vi "SPD.Measurments Single Point.vi"(5 "Current Progress":refnum<vi>, 6 "Overall Progress":refnum<vi>, 7 "Continue":refnum<vi>, 8 "Error In":errorcluster, 11 "SPD.Stand Ctrl in":T1={"spdDeviceSession"={"spdRef"=0, "connected"=FALSE, "spdName"="", "specification"={"diod case"=enum."default", "type"=enum."Unknown", "frequency"=enum."Unknown"}, "hidSPD.Controller"={"TSet"=0.0, "HV_bias"=0.0, "DDS_stb_code"=0}, "hidSPD.Sturtup Values"={"TSet"=0.0, "HV_bias"=0.0, "DDS_stb_code"=0}}, "DevBSession"={"DevBRef"="", "connected"=FALSE}, "FreqCSession"={"FreqCRef"="", "timeout"=0.0, "Gate"=0.0, "connected"=FALSE}, "8164BSession"={"Connection ID"=refnum, "Connected"=FALSE, "Info"="", "Slots Info"=[]}, "LeCroySession"={"LeCroySession"="", "connected"=FALSE}, "Events"={"DCRTest"=refnum, "Stop"=refnum}, "configFile"={"configFile ref"=refnum, "configFile path"=path "", "equipmentFile ref"=refnum}, "SPD.Meas Grid"={"DateTime"="", "DT"=[], "Insensitivity"=[], "Temprature"=[], "Stb_code"=[], "HV_Bias"=[]}, "SPD.Queues"={"state queue"=refnum}, "Console"=refnum} {"spdDeviceSession"."hidSPD.Sturtup Values"."HV_bias" format="%#_6p, V"; "spdDeviceSession"."hidSPD.Sturtup Values"."TSet" format="%#_6p, DegC"; "spdDeviceSession"."hidSPD.Controller"."HV_bias" format="%#_6p, V"; "spdDeviceSession"."hidSPD.Controller"."TSet" format="%#_6p, DegC"}) -> (0 "Error Out":errorcluster, 2 "pass":bool, 3 "SPD.Stand Ctrl out":T1={"spdDeviceSession"={"spdRef"=0, "connected"=FALSE, "spdName"="", "specification"={"diod case"=enum."default", "type"=enum."Unknown", "frequency"=enum."Unknown"}, "hidSPD.Controller"={"TSet"=0.0, "HV_bias"=0.0, "DDS_stb_code"=0}, "hidSPD.Sturtup Values"={"TSet"=0.0, "HV_bias"=0.0, "DDS_stb_code"=0}}, "DevBSession"={"DevBRef"="", "connected"=FALSE}, "FreqCSession"={"FreqCRef"="", "timeout"=0.0, "Gate"=0.0, "connected"=FALSE}, "8164BSession"={"Connection ID"=refnum, "Connected"=FALSE, "Info"="", "Slots Info"=[]}, "LeCroySession"={"LeCroySession"="", "connected"=FALSE}, "Events"={"DCRTest"=refnum, "Stop"=refnum}, "configFile"={"configFile ref"=refnum, "configFile path"=path "", "equipmentFile ref"=refnum}, "SPD.Meas Grid"={"DateTime"="", "DT"=[], "Insensitivity"=[], "Temprature"=[], "Stb_code"=[], "HV_Bias"=[]}, "SPD.Queues"={"state queue"=refnum}, "Console"=refnum} {"spdDeviceSession"."hidSPD.Sturtup Values"."HV_bias" format="%#_6p, V"; "spdDeviceSession"."hidSPD.Sturtup Values"."TSet" format="%#_6p, DegC"; "spdDeviceSession"."hidSPD.Controller"."HV_bias" format="%#_6p, V"; "spdDeviceSession"."hidSPD.Controller"."TSet" format="%#_6p, DegC"})   [LabVIEW 2018]
uses:
  Instruments/KC705 DevBoard/typedefs/DevB.Session.ctl
  Instruments/KeySight 53230A/typedefs/FreqC.Session.ctl
  Instruments/KeySight 8164B/KeySight 8164B LAN InstrLib/typedefs/KeySight 8164B control.ctl
  Instruments/KeySight 8164B/KeySight 8164B LAN InstrLib.lvlib
  Instruments/LeCroy SDA830/typedefs/LeCroy.Session.ctl
  typedefs/SPD.Events.ctl
  <vilib>/Utility/config.llb/Config Data RefNum.ctl
  <vilib>/Utility/config.llb/NI_LVConfig.lvlib
  ConfigFile/SPD.Config File ctrl.ctl
  typedefs/SPD.Meas Grid.ctl
  typedefs/SPD.Stand state.ctl
  typedefs/SPD.Queues.ctl
  Instruments/SPD HID Interface/hidSPDLibForLabView/LibVIs/hidSPD Controls/hidSPD Controller.ctl
  Instruments/SPD HID Interface/hidSPDLibForLabView/hidSPDLibForLabView.lvlib
  Instruments/SPD HID Interface/hidSPDLibForLabView/LibVIs/hidSPD Controls/hidSPD SPD Type.ctl
  Instruments/SPD HID Interface/hidSPDLibForLabView/LibVIs/hidSPD Controls/hidSPD Device Session.ctl
  typedefs/SPD.Stand Ctrl.ctl
  Instruments/SPD HID Interface/hidSPDLibForLabView/LibVIs/hidSPD Controls/hidSPD SPD Diod Case.ctl
  Instruments/SPD HID Interface/hidSPDLibForLabView/LibVIs/hidSPD Controls/hidSPD.STB Frequency.ctl
  Instruments/SPD HID Interface/hidSPDLibForLabView/LibVIs/hidSPD Controls/hidSPD.SPD specification.ctl
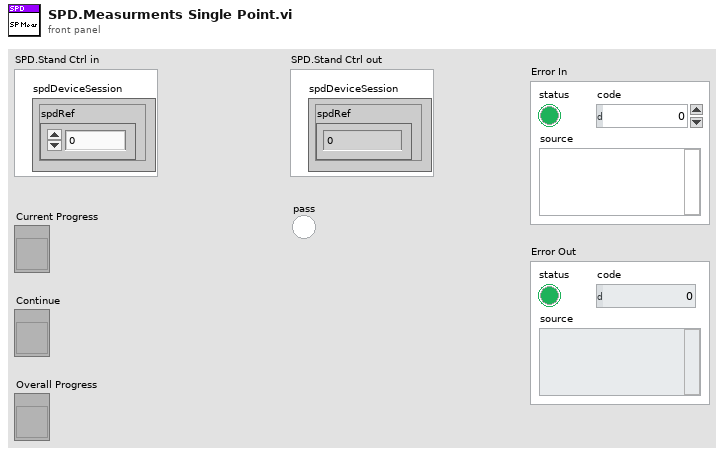
[diagram p1: front panel]
types:
  T1 = typedef "SPD.Stand Ctrl.ctl" = cluster{"spdDeviceSession":T2, "DevBSession":T8, "FreqCSession":T9, "8164BSession":T10, "LeCroySession":T11, "Events":T12, "configFile":T13, "SPD.Meas Grid":T15, "SPD.Queues":T16, "Console":refnum<vi>}
  T2 = typedef "hidSPDLibForLabView.lvlib/hidSPD Device Session.ctl" = cluster{"spdRef":u64, "connected":bool, "spdName":string, "specification":T3, "hidSPD.Controller":T7, "hidSPD.Sturtup Values":T7}
  T3 = typedef "hidSPDLibForLabView.lvlib/hidSPD.SPD specification.ctl" = cluster{"diod case":T4, "type":T5, "frequency":T6}
  T4 = typedef "hidSPDLibForLabView.lvlib/hidSPD SPD Diod Case.ctl" = enum16{"Unknown", "default", "butterfly"}
  T5 = typedef "hidSPDLibForLabView.lvlib/hidSPD SPD Type.ctl" = enum16{"Unknown", "Free Run", "Gate"}
  T6 = typedef "hidSPDLibForLabView.lvlib/hidSPD.STB Frequency.ctl" = enum16{"Unknown", "312", "1250"}
  T7 = typedef "hidSPDLibForLabView.lvlib/hidSPD Controller.ctl" = cluster{"TSet":sgl, "HV_bias":sgl, "DDS_stb_code":u16}
  T8 = typedef "DevB.Session.ctl" = cluster{"DevBRef":refnum<visa-resource-name>, "connected":bool}
  T9 = typedef "FreqC.Session.ctl" = cluster{"FreqCRef":refnum<visa-resource-name>, "timeout":dbl, "Gate":dbl, "connected":bool}
  T10 = typedef "KeySight 8164B LAN InstrLib.lvlib/KeySight 8164B control.ctl" = cluster{"Connection ID":refnum<k5>, "Connected":bool, "Info":string, "Slots Info":string[]}
  T11 = typedef "LeCroy.Session.ctl" = cluster{"LeCroySession":refnum<visa-resource-name>, "connected":bool}
  T12 = typedef "SPD.Events.ctl" = cluster{"DCRTest":refnum<user-event>, "Stop":refnum<user-event>}
  T13 = typedef "SPD.Config File ctrl.ctl" = cluster{"configFile ref":T14, "configFile path":path, "equipmentFile ref":T14}
  T14 = typedef "NI_LVConfig.lvlib/Config Data RefNum.ctl" = refnum<k1>
  T15 = typedef "SPD.Meas Grid.ctl" = cluster{"DateTime":string, "DT":dbl[], "Insensitivity":dbl[], "Temprature":dbl[], "Stb_code":dbl[], "HV_Bias":dbl[][][][]}
  T16 = typedef "SPD.Queues.ctl" = cluster{"state queue":refnum<queue>}
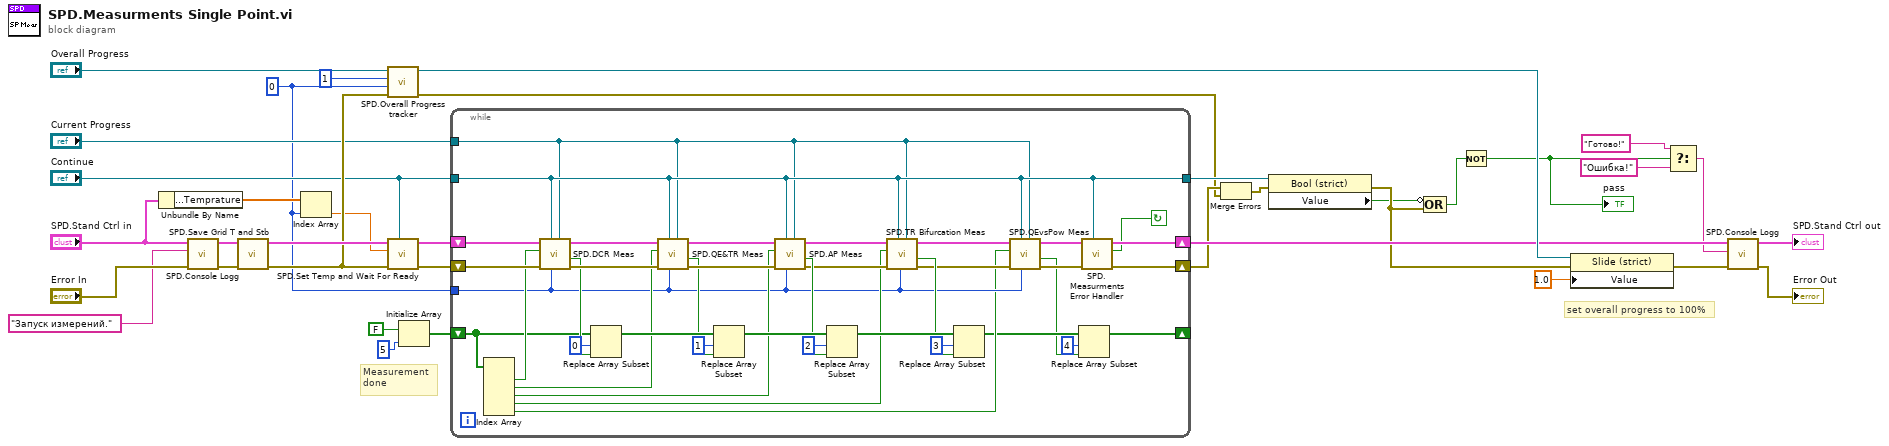
[diagram p0: block diagram]
diagram:
  w2 = 0
  # "Measurement\ndone"
  # "set overall progress to 100%"
  n1 = Unbundle By Name("SPD.Stand Ctrl in") -> ("SPD.Meas Grid.Temprature"=w3:dbl[])
  n2 = call "SPD.Console Logg.vi"("Error In"="Error In", "console Log"="Запуск измерений.", "SPD.Stand Ctrl in"="SPD.Stand Ctrl in") -> ("Error Out"=w26:errorcluster, "SPD.Stand Ctrl out"=w27:T1)  [unwired: 7 in]
  n3 = call "SPD.Save Grid T and Stb.vi"("Error In"=w26, "SPD.Stand Ctrl in"=w27) -> ("Error Out"=w35:errorcluster, "SPD.Stand Ctrl out"=w36:T1)  [unwired: 8 in]
  n4 = Index Array(array=w3, index=w2) -> (element=w1:dbl)
  n5 = call "SPD.Overall Progress tracker.vi"("Error In"=w35, "Num of temps"=w2, "Current temprature index"=1, "Slide in"="Overall Progress") -> ("Error Out"=w5:errorcluster, "Slide out"=w31:refnum<vi>)  [unwired: 6 in]
  n6 = call "SPD.Set Temp and Wait For Ready.vi"("Continue"="Continue", "Error In"=w35, "Tset"=w1, "SPD.Stand Ctrl in"=w36) -> ("Error Out"=w14:errorcluster, "SPD.Stand Ctrl out"=w15:T1)  [unwired: 6 in]
  n7 = Initialize Array(FALSE, 5 ("dimension size")) -> (w11:bool[])
  n8 = while {
    tunnel: w2 -> [w43]
    tunnel: "Current Progress" -> [w45]
    tunnel: "Continue" -> [w46]
    shift-right: [w63] -> w21
    shift-left: w15 -> [w54]
    shift-right: [w62] -> w9
    shift-left: w14 -> [w55]
    shift-right: [w39] -> _
    shift-left: w11 -> [w52]
    tunnel: [w46] -> w10
    stop <- w61 continue-if-true
    n9 = Index Array(array=w52) -> (element #1=w53:bool, element #2=w51:bool, element #3=w50:bool, element #4=w49:bool, element #5=w42:bool)  [unwired: 5 in]
    n10 = call "SPD.DCR Meas.vi"("Progress"=w45, "Temperature index"=w43, "Continue"=w46, "Error In"=w55, "Already done"=w53, "SPD.Stand Ctrl in"=w54) -> ("Error Out"=w74:errorcluster, "pass"=w71:bool, "SPD.Stand Ctrl out"=w75:T1)  [unwired: 2 in, 1 out]
    n11 = Replace Array Subset(array=w52, new element=w71, index=0) -> (w69:bool[])
    n12 = call "SPD.QE&TR Meas.vi"("Progress"=w45, "Temperature index"=w43, "Continue"=w46, "Error In"=w74, "Already done"=w51, "SPD.Stand Ctrl in"=w75) -> ("Error Out"=w72:errorcluster, "pass"=w67:bool, "SPD.Stand Ctrl out"=w73:T1)  [unwired: 2 in, 1 out]
    n13 = Replace Array Subset(array=w69, new element=w67, index=1) -> (w65:bool[])
    n14 = call "SPD.AP Meas.vi"("Progress"=w45, "Temperature index"=w43, "Continue"=w46, "Error In"=w72, "Already done"=w50, "SPD.Stand Ctrl in"=w73) -> ("Error Out"=w59:errorcluster, "pass"=w64:bool, "SPD.Stand Ctrl out"=w60:T1)  [unwired: 2 in, 1 out]
    n15 = Replace Array Subset(array=w65, new element=w64, index=2) -> (w57:bool[])
    n16 = call "SPD.TR Bifurcation Meas.vi"("Progress"=w45, "Temperature index"=w43, "Continue"=w46, "Error In"=w59, "Already done"=w49, "SPD.Stand Ctrl in"=w60) -> ("Error Out"=w47:errorcluster, "pass"=w56:bool, "SPD.Stand Ctrl out"=w48:T1)  [unwired: 2 in, 1 out]
    n17 = Replace Array Subset(array=w57, new element=w56, index=3) -> (w40:bool[])
    n18 = call "SPD.QEvsPow Meas.vi"("Progress"=w45, "Temperature index"=w43, "Continue"=w46, "Error In"=w47, "Already done"=w42, "SPD.Stand Ctrl in"=w48) -> ("Error Out"=w44:errorcluster, "pass"=w38:bool, "SPD.Stand Ctrl out"=w37:T1)  [unwired: 2 in, 1 out]
    n19 = Replace Array Subset(array=w40, new element=w38, index=4) -> (w39:bool[])
    n20 = call "SPD.Measurments Error Handler.vi"("Continue"=w46, "Error In"=w44, "SPD.Stand Ctrl in"=w37) -> ("Error Out"=w62:errorcluster, "Re-Measure"=w61:bool, "SPD.Stand Ctrl out"=w63:T1)  [unwired: 6 in]
  }
  n21 = Merge Errors(w9, w5) -> (w6:errorcluster)
  n22 = property class="Bool (strict)"(reference=w10, error in=w6) -> (error out=w17:errorcluster, "Value"=w8:bool)  [unwired: 1 out]
  n23 = Compound Arithmetic op=OR(invert w8, w17) -> (w7:bool)
  n24 = Not(x=w7) -> (.not. x?=w22:bool)
  "pass" <- w22
  n25 = property on="Property Node" class="Slide (strict)"(reference=w31, error in=w17, "Value"=1.0) -> (error out=w16:errorcluster)  [unwired: 1 out]
  n26 = Select(t="Готово!" ("Report"), s=w22, f="Ошибка!") -> (s? t:f=w20:string)
  n27 = call "SPD.Console Logg.vi"("Error In"=w16, "console Log"=w20, "SPD.Stand Ctrl in"=w21) -> ("Error Out"=→"Error Out":errorcluster, "SPD.Stand Ctrl out"=→"SPD.Stand Ctrl out":T1)  [unwired: 7 in]
